vi "Run.vi"(8 "error in (no error)":errorcluster, 11 "LCR-Measurement in":refnum<class "LCR-Meas.lvclass">) -> (0 "error out":errorcluster, 1 "Parameters":cluster{"Name":string, "Value":string}[](array[cluster]), 2 "Canceled":bool, 3 "LCR-Measurement out":refnum<class "LCR-Meas.lvclass">)   [LabVIEW 2020, in "LCR-Meas.lvclass"]
doc: "This is the main test vi. It is here that the test is implemented."
uses:
  LCR-Meas.lvclass
  C:/Sandbox/Git_Sandbox/WiSpry Test Framework source code (LV20)/WiSpry Test Framework/Measurements/Measurement.lvclass
  Controls/Run States.ctl
  Instruments/LCR Meter/Controls/Function.ctl
  Devices/Controls/Change setting mode enum.ctl
  Measurement.lvclass/Measurement.ctl
  XML Handler/Controls/Result Cluster.ctl
  Support VI/Update parameters (single).vi
  Support VI/Update parameters (array).vi
  Measurement.lvclass
  Instruments/LCR Meter/LCR Meter.lvclass
  Devices/Device.lvclass
  Devices/PIC-device/PIC-Device.lvclass
  XML Handler/XML Handler.lvclass
  Instruments/Power Supply/Power Supply.lvclass
  Instruments/Digital Multimeter/Digital Multimeter.lvclass
panel:
  out "Tab Control":enum32{"Page 1", "Page 2"}(tab)
  out "XY Graph":T1(graph)
  out "Waveform Chart":dbl[](graph)
  in  "Cancel Button":bool
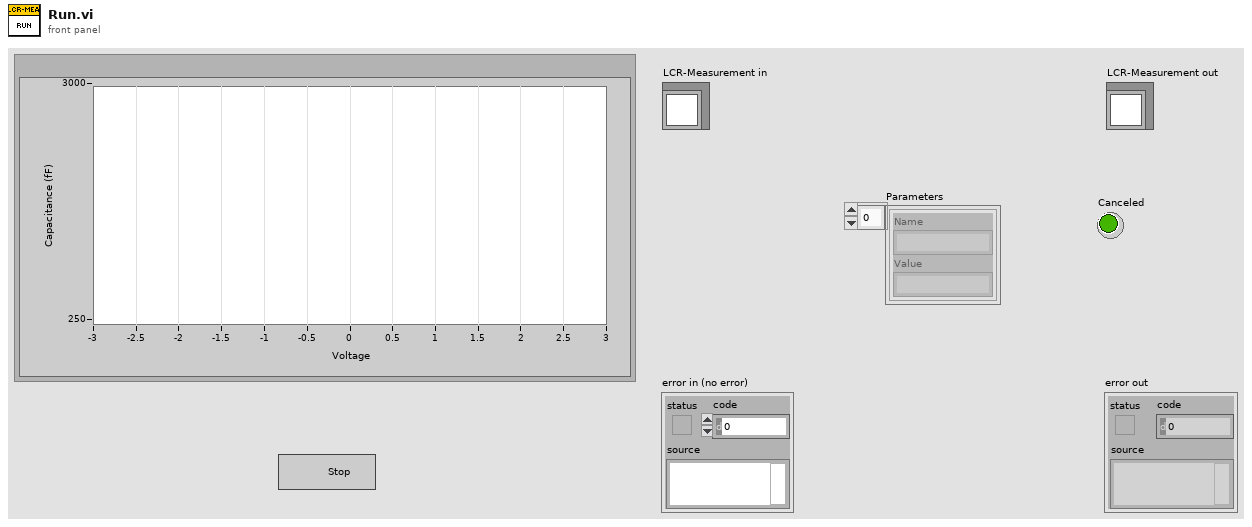
[diagram p1: front panel]
types:
  T1 = cluster{"Bias Voltages (V)":dbl[], "Capacitances (fF)":dbl[]}[]
  T2 = typedef "Measurement.lvclass/Run States.ctl" = enum16{"Init", "Set Device", "Read Environment", "Measure", "Done"}
  T3 = cluster{"Bias Voltages (V)":dbl[], "Capacitances (fF)":dbl[]}
  T4 = typedef "LCR Meter.lvclass/Function.ctl" = enum16{"Cp-D", "Cp-Q", "Cp-G", "Cp-Rp", "Cs-D", "Cs-Q", "Cs-Rs", "Lp-D", "Lp-Q", "Lp-G", "Lp-Rp", "Lp-Rdc", "Ls-D", "Ls-Q", "Ls-Rs", "Ls-Rdc", "R-X", "Z-thd", "Z-thr", "G-B", "Y-thd", "Y-thr", "Vdc-Idc"}
  T5 = typedef "PIC-Device.lvclass/Change setting mode enum.ctl" = enum16{"Init", "Next", "Reset"}
  T6 = typedef "XML Handler.lvclass/Result Cluster.ctl" = cluster{"Name":string, "Value":string}
  T7 = cluster{"Value":string, "Capacitance (fF)":string}
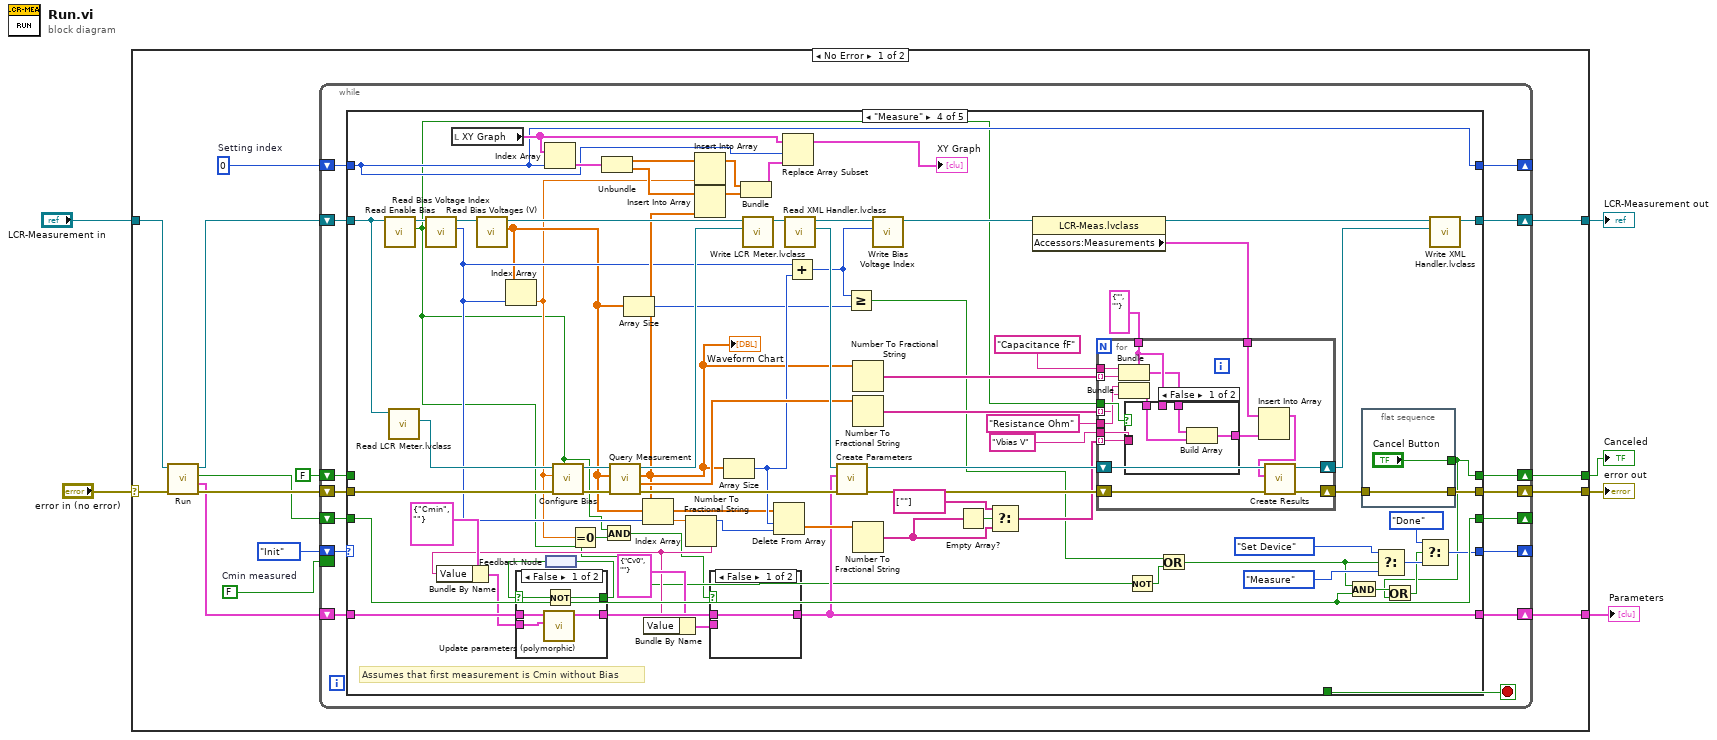
[diagram p0: block diagram]
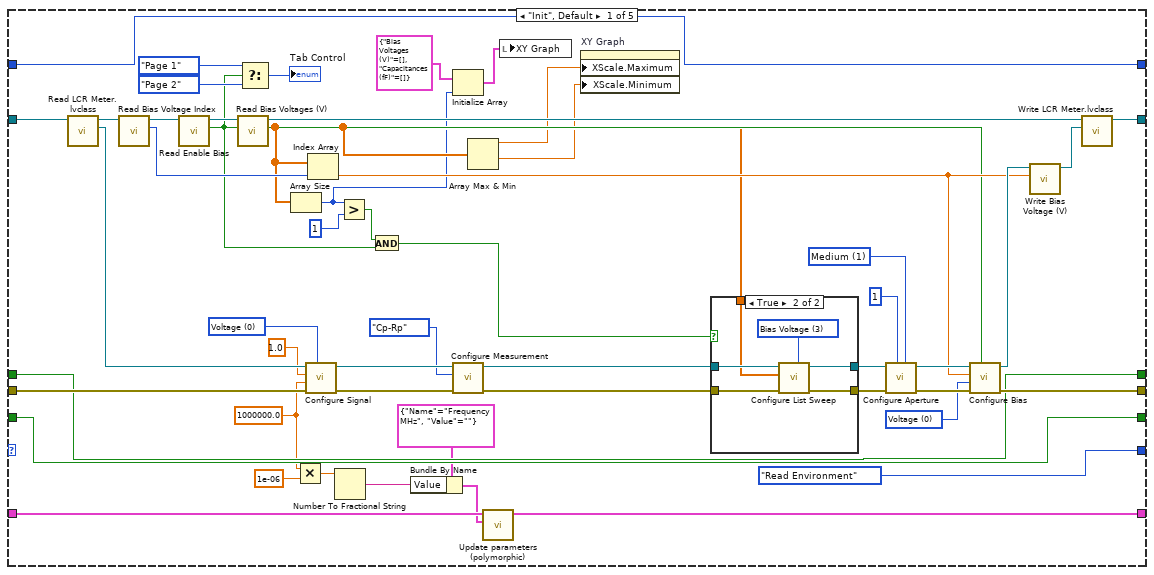
[diagram p2: hidden frame]
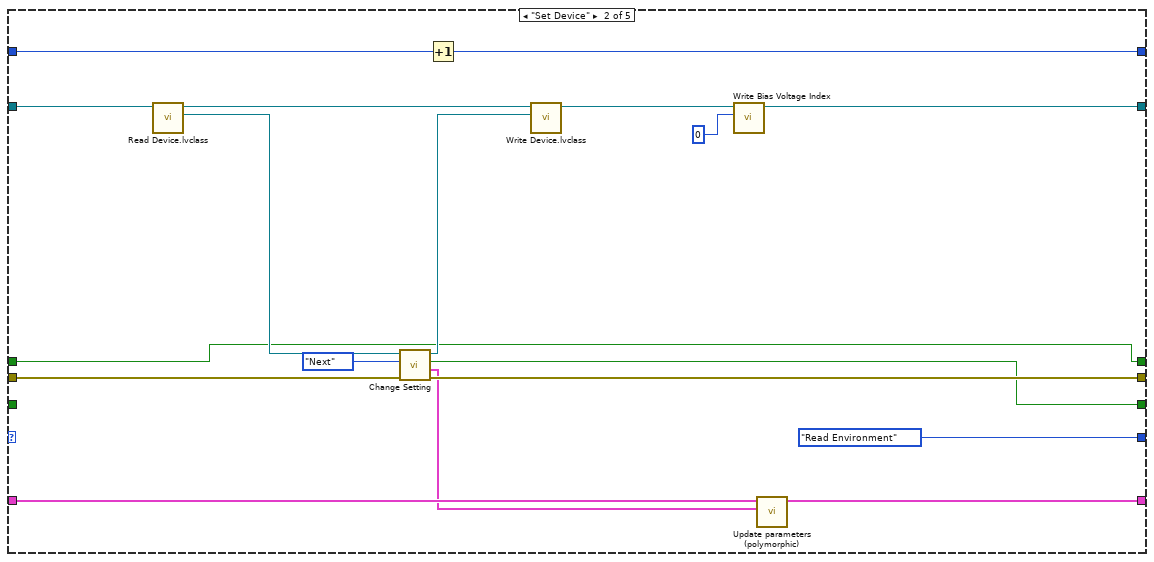
[diagram p4: hidden frame]
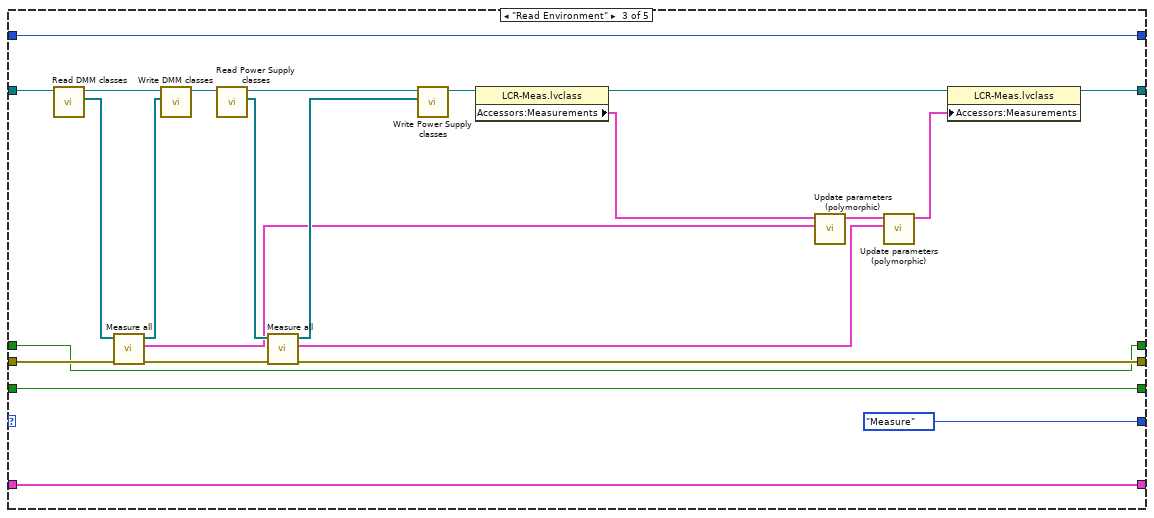
[diagram p5: hidden frame]
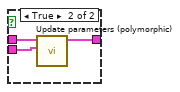
[diagram p6: hidden frame]
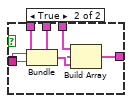
[diagram p8: hidden frame]
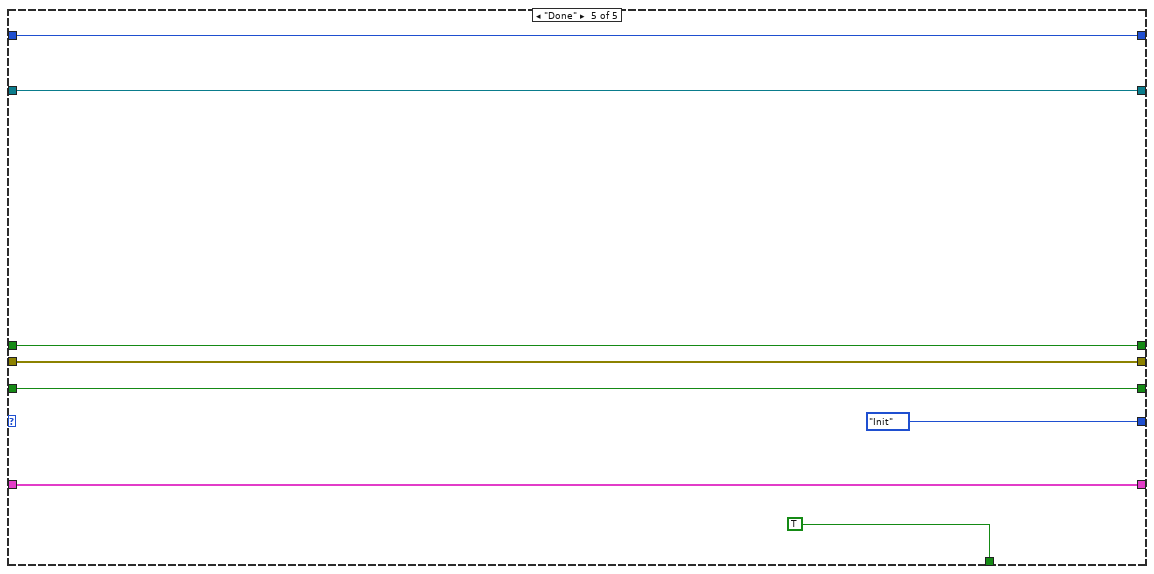
[diagram p9: hidden frame]
diagram:
  n1 = case shown="No Error" "error in (no error)" {
    selector: "error in (no error)" -> [w20 w263]
    tunnel: "LCR-Measurement in" -> [w19 w262]
    tunnel: [w17 w263] -> w4
    tunnel: [w15 w262] -> w3
    tunnel: [w14 _] -> w2
    tunnel: [w13 _] -> w1
    frame No Error {
      w7 = 0  # Setting index
      w8 = FALSE  # Cmin measured
      n2 = call-parent "Run.vi"("error in (no error)"=w20, "Measurements in"=w19) -> ("error out"=w18:errorcluster, "Parameters"=w9:cluster{"Name":string, "Value":string}[], "Canceled"=w11:bool, "Measurements out"=w16:refnum<class "LCR-Meas.lvclass">)  [unwired: 6 in]
      n3 = while {
        shift-right: [w33] -> w17
        shift-left: w18 -> [w34]
        shift-right: [w32] -> w15
        shift-left: w16 -> [w31]
        shift-right: [w29] -> _
        shift-left: Run_States."Init" ("Run states") -> [w35]
        shift-right: [w27] -> w13
        shift-left: w9 -> [w28]
        shift-right: [w26] -> _
        shift-left: w11 -> [w25]
        shift-right: [w23] -> w14
        shift-left: FALSE ("Cancel Button") -> [w24]
        border: w8 -> [_]
        shift-right: [w21] -> _
        shift-left: w7 -> [w22]
        stop <- w30 stop-if-true
        n4 = case shown="\"Measure\"" w35 {
          tunnel: w34 -> [w79 w112 w129 w186 w261]
          tunnel: [w78 w111 w125 w174 w261] -> w33
          tunnel: [w76 w100 w120 w206 w260] -> w32
          tunnel: w31 -> [w77 w105 w136 w192 w260]
          tunnel: [_ _ _ _ TRUE] -> w30
          tunnel: [Run_States."Read Environment" ("Run states") Run_States."Read Environment" ("Run states") Run_States."Measure" ("Run states") w209 Run_States."Init" ("Run states")] -> w29
          tunnel: [w51 w101 w121 w172 w255] -> w23
          tunnel: w28 -> [w50 w108 w119 w168 w256]
          tunnel: [w49 w106 w119 w145 w256] -> w27
          tunnel: [w52 w103 w135 w211 w257] -> w26
          tunnel: w25 -> [w52 _ w135 w211 w257]
          tunnel: w24 -> [w51 w101 w121 _ w255]
          tunnel: w22 -> [w36 w97 w114 w153 w254]
          tunnel: [w36 w96 w114 w153 w254] -> w21
          frame "Init", Default {
            w61 = u16 0 items=["Voltage", "Current"] ("DC Bias Type (0: Voltage)")
            w70 = u16 1 items=["Short", "Medium", "Long"] ("Measurement Time (1: Medium)")
            w47 = 1000000.0 ("Signal Frequency (1000 Hz)")
            w74 = u16 0 items=["Voltage", "Current"] ("Signal Type (0: Voltage)")
            n5 = call-dynamic "Read LCR Meter.lvclass.vi"("LCR-Measurement in"=w77) -> ("LCR Meter.lvclass"=w75:refnum<class "LCR Meter.lvclass">, "LCR-Measurement out"=w65:refnum<class "LCR-Meas.lvclass">)  [unwired: 9 in]
            n6 = call-dynamic "Read Bias Voltage Index.vi"("LCR-Measurement in"=w65) -> ("Bias Voltage Index"=w63:i32, "LCR-Measurement out"=w64:refnum<class "LCR-Meas.lvclass">)  [unwired: 9 in]
            n7 = call-dynamic "Read Enable Bias.vi"("LCR-Measurement in"=w64) -> ("Enable Bias"=w54:bool, "LCR-Measurement out"=w67:refnum<class "LCR-Meas.lvclass">)  [unwired: 9 in]
            n8 = call-dynamic "Read Bias Voltages (V).vi"("LCR-Measurement in"=w67) -> ("Bias Voltages (V)"=w42:dbl[], "LCR-Measurement out"=w66:refnum<class "LCR-Meas.lvclass">)  [unwired: 9 in]
            n9 = Select(t=enum32{"Page 1", "Page 2"}."Page 1" ("Tab Control"), s=w54, f=enum32{"Page 1", "Page 2"}."Page 2" ("Tab Control")) -> (s? t:f=→"Tab Control":enum32{"Page 1", "Page 2"})
            n10 = Array Size(array=w42) -> (size(s)=w38:i32)
            n11 = Multiply(x=w47, y=1e-06) -> (x*y=w45:dbl)
            n12 = call-dynamic "Configure Signal.vi"("Signal Type (0: Voltage)"=w74, "error in (no error)"=w79, "Signal Frequency (1 MHz)"=w47, "Signal Level (1.0 V)"=1.0, "LCR Meter in"=w75) -> ("error out"=w86:errorcluster, "LCR Meter out"=w87:refnum<class "LCR Meter.lvclass">)  [unwired: 5 in]
            n13 = Index Array(array=w42, index=w63) -> (element=w62:dbl)
            n14 = Number To Fractional String(number=w45) -> (F-format string=w44:string)  [unwired: 3 in]
            n15 = Greater?(x=w38, y=1) -> (0:w58:bool)
            n16 = And(x=w58, y=w54) -> (x .and. y?=w60:bool)
            n17 = Bundle By Name(cluster=cluster{"Name":string, "Value":string} {"Name"="Frequency MHz", "Value"=""} ("New Parameter"), "Value"=w44) -> (w43:cluster{"Name":string, "Value":string})
            n18 = Initialize Array(T3 {"Bias Voltages (V)"=[], "Capacitances (fF)"=[]} ("XY Graph"), w38) -> (w37:T1)
            n19 = call-dynamic "Configure Measurement.vi"("error in (no error)"=w86, "Function (0: Cp-D)"=Function."Cp-Rp", "LCR Meter in"=w87) -> ("error out"=w84:errorcluster, "LCR Meter out"=w85:refnum<class "LCR Meter.lvclass">)  [unwired: 7 in]
            n20 = Array Max & Min(array=w42) -> (max value=w41:dbl, min value=w40:dbl)  [unwired: 2 out]
            n21 = call-poly "Update parameters (polymorphic).vi"("New Parameter"=w43, "Parameters"=w50) -> ("Parameters Out"=w49:cluster{"Name":string, "Value":string}[])  [unwired: 9 in]
            n22 = local write "XY Graph"(w37) -> ()
            n23 = property on="XY Graph" class="XYGraph (strict)"("XScale.Maximum"=w41, "XScale.Minimum"=w40) -> ()  [unwired: 2 in, 2 out]
            n24 = case shown="True" w60 {
              tunnel: w85 -> [w89 w95]
              tunnel: w84 -> [w88 w94]
              tunnel: [w89 w93] -> w83
              tunnel: [w88 w92] -> w82
              tunnel: w42 -> [_ w91]
              frame False {
              }
              frame True {
                w90 = u16 3 items=["Frequency", "Voltage", "Current", "Bias Voltage", "Bias Current", "DC Source Voltage"] ("Sweep Function A (0: Frequency)")
                n25 = call-dynamic "Configure List Sweep.vi"("Sweep Function A (0: Frequency)"=w90, "error in (no error)"=w94, "Sweep Point Array"=w91, "LCR Meter in"=w95) -> ("error out"=w92:errorcluster, "LCR Meter out"=w93:refnum<class "LCR Meter.lvclass">)  [unwired: 6 in]
              }
            }
            n26 = call-dynamic "Configure Aperture.vi"("Measurement Time (1: Medium)"=w70, "Averaging Factor (1)"=1, "error in (no error)"=w82, "LCR Meter in"=w83) -> ("error out"=w80:errorcluster, "LCR Meter out"=w81:refnum<class "LCR Meter.lvclass">)  [unwired: 6 in]
            n27 = call-dynamic "Configure Bias.vi"("DC Bias State (F:Disable)"=w54, "error in (no error)"=w80, "DC Bias Type (0: Voltage)"=w61, "DC Bias Level (0.0 V)"=w62, "LCR Meter in"=w81) -> ("error out"=w78:errorcluster, "LCR Meter out"=w68:refnum<class "LCR Meter.lvclass">)  [unwired: 5 in]
            n28 = call-dynamic "Write Bias Voltage (V).vi"("Bias Voltage (V)"=w62, "LCR Meter in"=w68) -> ("LCR Meter out"=w69:refnum<class "LCR Meter.lvclass">)  [unwired: 9 in]
            n29 = call-dynamic "Write LCR Meter.lvclass.vi"("LCR Meter.lvclass"=w69, "LCR-Measurement in"=w66) -> ("LCR-Measurement out"=w76:refnum<class "LCR-Meas.lvclass">)  [unwired: 9 in]
          }
          frame "Set Device" {
            n30 = call "Read Device.lvclass.vi"("Measurements in"=w105) -> ("Device.lvclass"=w102:refnum<class "Device.lvclass">, "Measurements out"=w110:refnum<class "LCR-Meas.lvclass">)  [unwired: 9 in]
            n31 = call-dynamic "Change Setting.vi"("error in (no error)"=w112, "Change setting mode"=Change_setting_mode_enum."Next", "Device in"=w102) -> ("error out"=w111:errorcluster, "Changes"=w107:cluster{"Name":string, "Value":string}[], "Last setting"=w103:bool, "Device out"=w109:refnum<class "Device.lvclass">)  [unwired: 5 in]
            n32 = Increment(x=w97) -> (x+1=w96:i32)
            n33 = call "Write Device.lvclass.vi"("Device.lvclass"=w109, "Measurements in"=w110) -> ("Measurements out"=w99:refnum<class "LCR-Meas.lvclass">)  [unwired: 9 in]
            n34 = call-dynamic "Write Bias Voltage Index.vi"("Bias Voltage Index"=0, "LCR-Measurement in"=w99) -> ("LCR-Measurement out"=w100:refnum<class "LCR-Meas.lvclass">)  [unwired: 9 in]
            n35 = call-poly "Update parameters (polymorphic).vi"("New Parameters"=w107, "Parameters"=w108) -> ("Parameters Out"=w106:cluster{"Name":string, "Value":string}[])  [unwired: 9 in]
          }
          frame "Read Environment" {
            n36 = call-dynamic "Read DMM classes.vi"("Measurements in"=w136) -> ("DMM classes"=w126:refnum<class "Digital Multimeter.lvclass">[], "Measurements out"=w137:refnum<class "LCR-Meas.lvclass">)  [unwired: 9 in]
            n37 = call "Measure all.vi"("error in (no error)"=w129, "Digital Multimeters in"=w126) -> ("error out"=w128:errorcluster, "Measurements"=w124:T6[], "Digital Multimeters out"=w127:refnum<class "Digital Multimeter.lvclass">[])  [unwired: 5 in, 2 out]
            n38 = call-dynamic "Write DMM classes.vi"("DMM classes"=w127, "Measurements in"=w137) -> ("Measurements out"=w133:refnum<class "LCR-Meas.lvclass">)  [unwired: 9 in]
            n39 = call-dynamic "Read Power Supply classes.vi"("Measurements in"=w133) -> ("Power Supply classes"=w131:refnum<class "Power Supply.lvclass">[], "Measurements out"=w132:refnum<class "LCR-Meas.lvclass">)  [unwired: 9 in]
            n40 = call "Measure all.vi"("error in (no error)"=w128, "Power Supplies in"=w131) -> ("error out"=w125:errorcluster, "Measurements"=w122:T6[], "Power Supplies out"=w130:refnum<class "Power Supply.lvclass">[])  [unwired: 5 in, 2 out]
            n41 = call-dynamic "Write Power Supply classes.vi"("Power Supply classes"=w130, "Measurements in"=w132) -> ("Measurements out"=w117:refnum<class "LCR-Meas.lvclass">)  [unwired: 9 in]
            n42 = property class="LCR-Meas.lvclass"(reference=w117) -> (reference out=w116:refnum<class "LCR-Meas.lvclass">, "Accessors:Measurements"=w118:cluster{"Name":string, "Value":string}[])  [unwired: 1 in, 1 out]
            n43 = call-poly "Update parameters (polymorphic).vi"("New Parameters"=w124, "Parameters"=w118) -> ("Parameters Out"=w123:cluster{"Name":string, "Value":string}[])  [unwired: 9 in]
            n44 = call-poly "Update parameters (polymorphic).vi"("New Parameters"=w122, "Parameters"=w123) -> ("Parameters Out"=w115:cluster{"Name":string, "Value":string}[])  [unwired: 9 in]
            n45 = property class="LCR-Meas.lvclass"(reference=w116, "Accessors:Measurements"=w115) -> (reference out=w120:refnum<class "LCR-Meas.lvclass">)  [unwired: 1 in, 1 out]
          }
          frame "Measure" {
            # "Assumes that first measurement is Cmin without Bias"
            n46 = call-dynamic "Read Enable Bias.vi"("LCR-Measurement in"=w192) -> ("Enable Bias"=w139:bool, "LCR-Measurement out"=w169:refnum<class "LCR-Meas.lvclass">)  [unwired: 9 in]
            n47 = call-dynamic "Read LCR Meter.lvclass.vi"("LCR-Measurement in"=w192) -> ("LCR Meter.lvclass"=w183:refnum<class "LCR Meter.lvclass">)  [unwired: 9 in, 1 out]
            n48 = call-dynamic "Read Bias Voltage Index.vi"("LCR-Measurement in"=w169) -> ("Bias Voltage Index"=w152:i32, "LCR-Measurement out"=w171:refnum<class "LCR-Meas.lvclass">)  [unwired: 9 in]
            n49 = local read "XY Graph"() -> (w156:T1)
            n50 = call-dynamic "Read Bias Voltages (V).vi"("LCR-Measurement in"=w171) -> ("Bias Voltages (V)"=w149:dbl[], "LCR-Measurement out"=w170:refnum<class "LCR-Meas.lvclass">)  [unwired: 9 in]
            n51 = Index Array(array=w149, index=w152) -> (element=w141:dbl)
            n52 = Index Array(array=w156, index=w153) -> (element=w155:T3)
            n53 = feedback #1() -> (w167:bool)
            n54 = call-dynamic "Configure Bias.vi"("DC Bias State (F:Disable)"=w139, "error in (no error)"=w186, "DC Bias Level (0.0 V)"=w141, "LCR Meter in"=w183) -> ("error out"=w185:errorcluster, "LCR Meter out"=w184:refnum<class "LCR Meter.lvclass">)  [unwired: 6 in]
            n55 = Equal To 0?(x=w141) -> (x = 0?=w140:bool)
            n56 = Unbundle(w155) -> ("Bias Voltages (V)"=w162:dbl[], "Capacitances (fF)"=w161:dbl[])
            n57 = And(x=w139, y=w140) -> (x .and. y?=w138:bool)
            n58 = call-dynamic "Query Measurement.vi"("error in (no error)"=w185, "States"=w149, "LCR Meter in"=w184) -> ("error out"=w198:errorcluster, "Secondary results"=w189:dbl[], "Capacitances (fF)"=w160:dbl[], "LCR Meter out"=w202:refnum<class "LCR Meter.lvclass">)  [unwired: 5 in]
            "Waveform Chart" <- w160
            n59 = Array Size(array=w149) -> (size(s)=w148:i32)
            n60 = Index Array(array=w160) -> (element=w164:dbl)  [unwired: 1 in]
            n61 = Number To Fractional String(number=w164) -> (F-format string=w142:string)  [unwired: 3 in]
            n62 = Bundle By Name(cluster=cluster{"Name":string, "Value":string} {"Name"="Cmin", "Value"=""} ("Cluster"), "Value"=w142) -> (w163:cluster{"Name":string, "Value":string})
            n63 = case shown="False" w167 {
              selector: w167 -> [w220 w223]
              tunnel: w168 -> [w222 w224]
              tunnel: [w221 w224] -> w146
              tunnel: [w219 w223] -> w166
              tunnel: w163 -> [w218 _]
              frame False {
                n64 = call-poly "Update parameters (polymorphic).vi"("New Parameter"=w218, "Parameters"=w222) -> ("Parameters Out"=w221:cluster{"Name":string, "Value":string}[])  [unwired: 9 in]
                n65 = Not(x=w220) -> (.not. x?=w219:bool)
              }
              frame True {
              }
            }
            n66 = feedback-in #1(w166) -> ()
            n67 = Bundle By Name(cluster=cluster{"Name":string, "Value":string} {"Name"="Cv0", "Value"=""} ("Cluster"), "Value"=w142) -> (w143:cluster{"Name":string, "Value":string})
            n68 = Insert Into Array(array=w162, new element=w141) -> (w159:dbl[])  [unwired: 1 in]
            n69 = Insert Into Array(array=w161, new element=w160) -> (w158:dbl[])  [unwired: 1 in]
            n70 = case shown="False" w138 {
              tunnel: w146 -> [w214 w217]
              tunnel: [w214 w216] -> w145
              tunnel: w143 -> [_ w215]
              frame False {
              }
              frame True {
                n71 = call-poly "Update parameters (polymorphic).vi"("New Parameter"=w215, "Parameters"=w217) -> ("Parameters Out"=w216:cluster{"Name":string, "Value":string}[])  [unwired: 9 in]
              }
            }
            n72 = Array Size(array=w160) -> (size(s)=w182:i32)
            n73 = Bundle("Bias Voltages (V)"=w159, "Capacitances (fF)"=w158) -> (w154:T3)  [unwired: 1 in]
            n74 = call-dynamic "Write LCR Meter.lvclass.vi"("LCR Meter.lvclass"=w202, "LCR-Measurement in"=w170) -> ("LCR-Measurement out"=w201:refnum<class "LCR-Meas.lvclass">)  [unwired: 9 in]
            n75 = Delete From Array(array=w149, length=w182, index=w152) -> (deleted portion=w181:dbl[])  [unwired: 1 out]
            n76 = Replace Array Subset(array=w156, new element=w154, index=w153) -> (→"XY Graph":T1)
            n77 = call "Read XML Handler.lvclass.vi"("Measurements in"=w201) -> ("XML Handler.lvclass"=w204:refnum<class "XML Handler.lvclass">, "Measurements out"=w205:refnum<class "LCR-Meas.lvclass">)  [unwired: 9 in]
            n78 = Add(x=w152, y=w182) -> (x+y=w150:i32)
            n79 = call "Create Parameters.vi"("error in (no error)"=w198, "Parameters"=w145, "XML Handler in"=w204) -> ("error out"=w199:errorcluster, "XML Handler out"=w207:refnum<class "XML Handler.lvclass">)  [unwired: 7 in]
            n80 = Greater Or Equal?(x=w150, y=w148) -> (x >= y?=w147:bool)
            n81 = Number To Fractional String(number=w160) -> (F-format string=w195:string[])  [unwired: 3 in]
            n82 = Number To Fractional String(number=w189) -> (F-format string=w188:string[])  [unwired: 3 in]
            n83 = Number To Fractional String(number=w181) -> (F-format string=w151:string[])  [unwired: 3 in]
            n84 = call-dynamic "Write Bias Voltage Index.vi"("Bias Voltage Index"=w150, "LCR-Measurement in"=w205) -> ("LCR-Measurement out"=w180:refnum<class "LCR-Meas.lvclass">)  [unwired: 9 in]
            n85 = Empty Array?(array=w151) -> (empty?=w177:bool)
            n86 = Select(t=string[] [""], s=w177, f=w151) -> (s? t:f=w175:string[])
            n87 = property class="LCR-Meas.lvclass"(reference=w180) -> (reference out=w179:refnum<class "LCR-Meas.lvclass">, "Accessors:Measurements"=w178:cluster{"Name":string, "Value":string}[])  [unwired: 1 in, 1 out]
            n88 = for {
              shift-right: [w242] -> w203
              shift-left: w207 -> [w243]
              tunnel: T6 {"Name"="", "Value"=""} ("Result Cluster") -> [w241]
              shift-right: [w239] -> w173
              shift-left: w199 -> [w240]
              tunnel: "Capacitance fF" ("Value") -> [w238]
              tunnel: "Vbias V" ("Value") -> [w237]
              tunnel: w195 -> [w233] mode=indexing
              tunnel: w175 -> [w236] mode=indexing
              tunnel: w139 -> [w235]
              tunnel: w188 -> [w231] mode=indexing
              tunnel: "Resistance Ohm" ("Value") -> [w232]
              tunnel: w178 -> [w227]
              n89 = Bundle(cluster=w241, "Name"=w238, "Value"=w233) -> (w234:T6)
              n90 = Bundle("Value"=w232, "Capacitance (fF)"=w231) -> (w230:T7)  [unwired: 1 in]
              n91 = case shown="False" w235 {
                tunnel: w241 -> [_ w250]
                tunnel: w237 -> [_ w253]
                tunnel: w236 -> [_ w252]
                tunnel: w234 -> [w246 w249]
                tunnel: [w245 w248] -> w229
                tunnel: w230 -> [w244 w247]
                frame False {
                  n92 = Build Array(w246, w244) -> (w245:T6[])
                }
                frame True {
                  n93 = Bundle(cluster=w250, "Name"=w253, "Value"=w252) -> (w251:T6)
                  n94 = Build Array(w249, w247, w251) -> (w248:T6[])
                }
              }
              n95 = Insert Into Array(array=w227, new element=w229) -> (w228:cluster{"Name":string, "Value":string}[])  [unwired: 1 in]
              n96 = call "Create Results.vi"("error in (no error)"=w240, "Results"=w228, "XML Handler in"=w243) -> ("error out"=w239:errorcluster, "XML Handler out"=w242:refnum<class "XML Handler.lvclass">)  [unwired: 7 in]
            }
            n97 = Not(x=w139) -> (.not. x?=w190:bool)
            n98 = Or(x=w147, y=w190) -> (x .or. y?=w191:bool)
            n99 = And(x=w191, y=w211) -> (x .and. y?=w194:bool)
            n100 = flat-sequence {
              tunnel: [w226] -> w174
              tunnel: w173 -> [w226]
              tunnel: ["Cancel Button"] -> w172
              frame #0 {
              }
            }
            n101 = Select(t=Run_States."Set Device" ("Run states"), s=w191, f=Run_States."Measure" ("Run states")) -> (s? t:f=w210:T2)
            n102 = Or(x=w194, y=w172) -> (x .or. y?=w193:bool)
            n103 = Select(t=Run_States."Done" ("Run states"), s=w193, f=w210) -> (s? t:f=w209:T2)
            n104 = call "Write XML Handler.lvclass.vi"("XML Handler.lvclass"=w203, "Measurements in"=w179) -> ("Measurements out"=w206:refnum<class "LCR-Meas.lvclass">)  [unwired: 9 in]
          }
          frame "Done" {
          }
        }
      }
    }
    frame Error {
    }
  }
  "error out" <- w4
  "LCR-Measurement out" <- w3
  "Canceled" <- w2
  "Parameters" <- w1
